vi "SeCrTs-AO_Scale_Config.vi"(8 "error in (no error)":errorcluster, 10 "AO config":T1(array[cluster]), 11 "Refnum in":refnum<k21>) -> (0 "error out":errorcluster, 3 "Refnum out":refnum<k21>)   [LabVIEW 2022 SP3]
uses:
  <vilib>/DAQmx/create/channels.llb/DAQmx Create Channel (AO-Voltage-Basic).vi
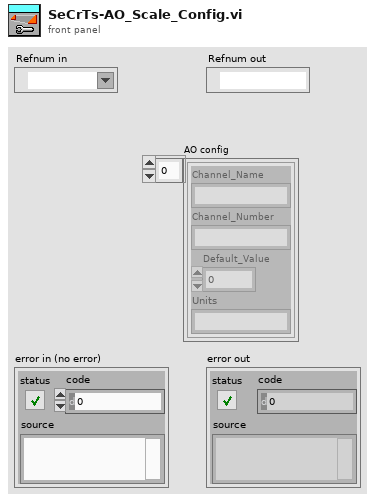
[diagram p1: front panel]
types:
  T1 = cluster{"Channel_Name":string, "Channel_Number":string, "Default_Value":dbl, "Units":string}[]
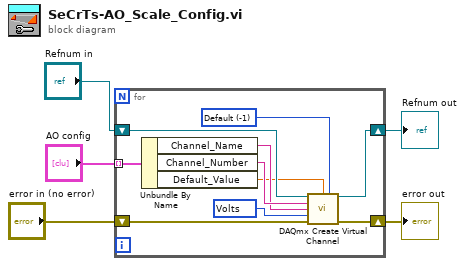
[diagram p0: block diagram]
diagram:
  n1 = for {
    shift-right: [w14] -> w2
    shift-left: "error in (no error)" -> [w8]
    tunnel: "AO config" -> [w12] mode=indexing
    shift-right: [w15] -> w3
    shift-left: "Refnum in" -> [w11]
    w6 = -1 items=["Default"=-1, "RSE"=10083, "Differential"=10106, "Pseudodifferential"=12529] ("output terminal configuration")
    w13 = 10348 items=["Volts"=10348, "From Custom Scale"=10065] ("units")
    n2 = Unbundle By Name(w12) -> ("Channel_Name"=w9:string, "Channel_Number"=w10:string, "Default_Value"=w7:dbl)
    n3 = call-poly <vilib>:"DAQmx Create Virtual Channel.vi"("task in"=w11, "minimum value"=w7, "output terminal configuration"=w6, "physical channels"=w10, "name to assign"=w9, "units"=w13, "error in"=w8) -> ("task out"=w15:refnum<k21>, "error out"=w14:errorcluster)  [unwired: 7 in]
  }
  "Refnum out" <- w3
  "error out" <- w2
